vi "Init Editor.vi"(9 "Update Preview":refnum<user-event>, 10 "Autocomplete Options":refnum<class "Shared Options.lvclass">, 11 "ElementEditorPanel in":refnum<class "ElementEditorPanel.lvclass">) -> (3 "ElementEditorPanel out":refnum<class "ElementEditorPanel.lvclass">)   [LabVIEW 2020, in "VolatusGUIControls.lvlib" / "ElementEditorPanel.lvclass"]
uses:
  ElementEditorPanel.lvclass
  ElementEditorPanel.lvclass/ElementEditorPanel.ctl
  lv-autocomplete/AutoComplete/Shared Options/Shared Options.lvclass
  VolatusGUIEditor/Update Preview Data.ctl
  VolatusGUIEditor/VolatusGUIEditor.lvlib
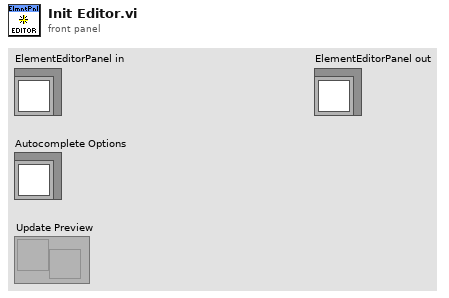
[diagram p1: front panel]
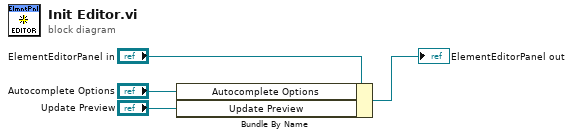
[diagram p0: block diagram]
diagram:
  n1 = Bundle By Name(cluster="ElementEditorPanel in", "Autocomplete Options"="Autocomplete Options", "Update Preview"="Update Preview") -> (→"ElementEditorPanel out":refnum<class "ElementEditorPanel.lvclass">)
